vi "Run Option.vi"(7 "Timeout":i32=-1, 11 "Car Wash Station Sequencer in":refnum<class "Car Wash Station Sequencer.lvclass">) -> (3 "Car Wash Station Sequencer out":refnum<class "Car Wash Station Sequencer.lvclass">, 5 "Timeout out":i32)   [LabVIEW 2016, in "CLD Exam - Car Wash.lvlib" / "Car Wash Station Sequencer.lvclass"]
uses:
  Car Wash Station Sequencer.lvclass
  D:/Repos/Stream/software/Mediator/Classes/Mediated Actor/Mediated Actor.lvclass
  Car Wash Station Sequencer.lvclass/Car Wash Station Sequencer.ctl
  Mediator/Classes/Message Interface/Message Interface.lvclass
  Car Wash Option Finished Event/Car Wash Option Finished.lvclass
  D:/Repos/Stream/software/Mediator/Classes/Message Interface/Message Interface.lvclass
  Mediator/Classes/Message Transport Queue/Message Transport Queue.lvclass
  Mediator/Classes/Mediated Actor/Mediated Actor.lvclass
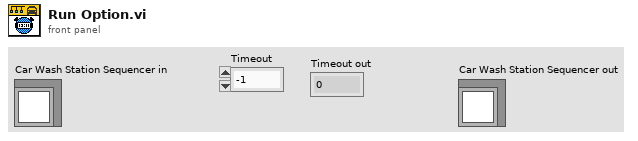
[diagram p1: front panel]
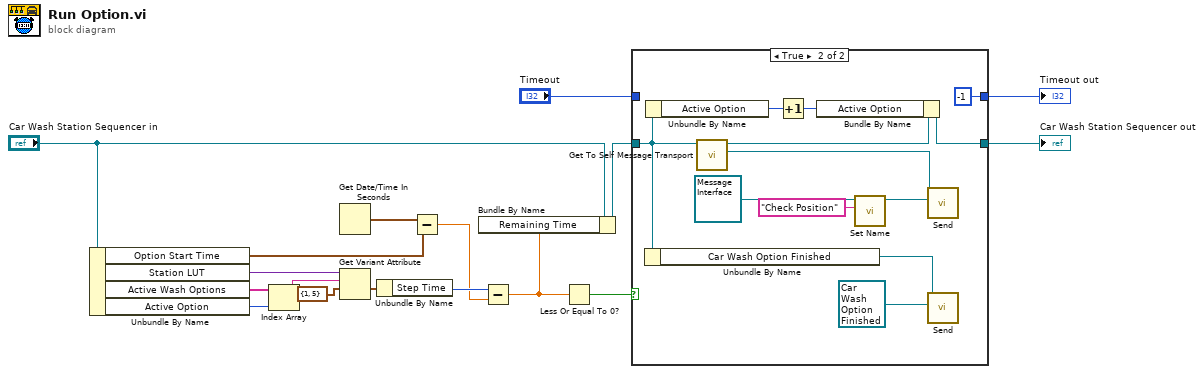
[diagram p0: block diagram]
diagram:
  n1 = Unbundle By Name("Car Wash Station Sequencer in") -> ("Option Start Time"=w6:timestamp, "Station LUT"=w15:variant, "Active Wash Options"=w17:string[], "Active Option"=w16:u8)
  n2 = Index Array(array=w17, index=w16) -> (element=w12:string)
  n3 = Get Date/Time In Seconds() -> (seconds since 1Jan1904=w11:timestamp)
  n4 = Get Variant Attribute(Variant=w15, name=w12, default value (empty Variant)=cluster{"Station":u8, "Step Time":u16} {"Station"=1, "Step Time"=5}) -> (value=w13:cluster{"Station":u8, "Step Time":u16})  [unwired: 1 in, 3 out]
  n5 = Unbundle By Name(w13) -> ("Step Time"=w10:u16)
  n6 = Subtract(x=w11, y=w6) -> (x-y=w9:dbl)
  n7 = Subtract(x=w10, y=w9) -> (x-y=w8:dbl)
  n8 = Bundle By Name(cluster="Car Wash Station Sequencer in", "Remaining Time"=w8) -> (w5:refnum<class "Car Wash Station Sequencer.lvclass">)
  n9 = Less Or Equal To 0?(x=w8) -> (x <= 0?=w3:bool)
  n10 = case shown="True" w3 {
    tunnel: w5 -> [w19 w24]
    tunnel: [w19 w22] -> w4
    tunnel: "Timeout" -> [w18 _]
    tunnel: [w18 -1 ("Timeout")] -> w1
    frame False {
    }
    frame True {
      n11 = Unbundle By Name(w24) -> ("Car Wash Option Finished"=w31:refnum<class "Message Transport Queue.lvclass">)
      n12 = Unbundle By Name(w24) -> ("Active Option"=w21:u8)
      n13 = call "Get To Self Message Transport.vi"("Mediated Actor in"=w24) -> ("To Self"=w30:refnum<class "Message Transport Queue.lvclass">, "Mediated Actor out"=w23:refnum<class "Car Wash Station Sequencer.lvclass">)  [unwired: 9 in]
      n14 = Increment(x=w21) -> (x+1=w20:u8)
      n15 = Bundle By Name(cluster=w23, "Active Option"=w20) -> (w22:refnum<class "Car Wash Station Sequencer.lvclass">)
      n16 = call "Set Name.vi"("Name"="Check Position", "Message Interface in"=refnum<class "Message Interface.lvclass"> refnum) -> ("Message Interface out"=w29:refnum<class "Message Interface.lvclass">)  [unwired: 8 in, 1 out]
      n17 = call-dynamic "Send.vi"("Message"=w29, "Message Transport Queue in"=w30) -> ()  [unwired: 7 in, 3 out]
      n18 = call-dynamic "Send.vi"("Message"=refnum<class "Car Wash Option Finished.lvclass"> refnum ("Car Wash Option Finished.lvclass"), "Message Transport Queue in"=w31) -> ()  [unwired: 7 in, 3 out]
    }
  }
  "Car Wash Station Sequencer out" <- w4
  "Timeout out" <- w1
